vi "GetValues.vi"(9 "error in":errorcluster) -> (1 "error out":errorcluster)   [LabVIEW 2017]
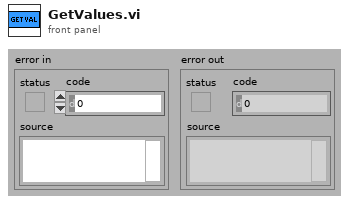
[diagram p1: front panel]
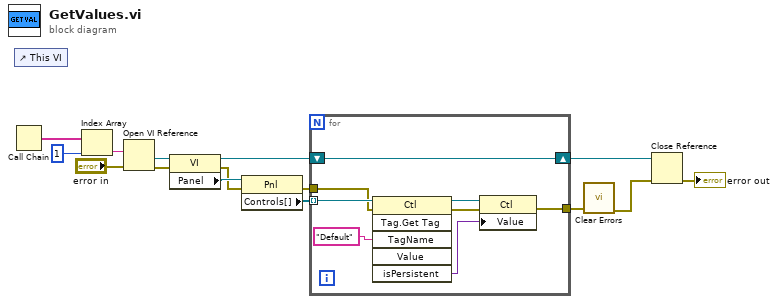
[diagram p0: block diagram]
diagram:
  n1 = Call Chain() -> (call chain=w15:string[])
  n2 = control-ref of="This VI"() -> ()  [unwired: 1 out]
  n3 = Index Array(array=w15, index=1) -> (element=w14:string)
  n4 = Open VI Reference(vi path=w14, error in (no error)="error in") -> (vi reference=w7:refnum<vi>, error out=w8:errorcluster)  [unwired: 4 in]
  n5 = property class="VI"(reference=w7, error in=w8) -> (reference out=w9:refnum<vi>, error out=w11:errorcluster, "Panel"=w12:refnum<vi>)
  n6 = property class="Pnl"(reference=w12, error in=w11) -> (error out=w6:errorcluster, "Controls[]"=w10:refnum<vi>[])  [unwired: 1 out]
  n7 = for {
    tunnel: w10 -> [w21] mode=indexing
    shift-right: [w22] -> w5
    shift-left: w9 -> [w22]
    tunnel: [w17] -> w3
    tunnel: w6 -> [w16]
    n8 = invoke class="Ctl" method="Tag.Get Tag"(reference=w21, error in=w16, "TagName"="Default" ("Tag Name")) -> (reference out=w20:refnum<vi>, error out=w18:errorcluster, "isPersistent"=w19:variant)  [unwired: 3 in, 3 out]
    n9 = property class="Ctl"(reference=w20, error in=w18, "Value"=w19) -> (error out=w17:errorcluster)  [unwired: 1 out]
  }
  n10 = call <vilib>:"Clear Errors.vi"("error in (no error)"=w3) -> ("error out"=w2:errorcluster)  [unwired: 5 in, 1 out]
  n11 = Close Reference(reference=w5, error in (no error)=w2) -> (error out=→"error out":errorcluster)
